vi "Copy attachment to data folder.vi"(10 "Str Refnum":refnum<vi>, 11 "Path in":refnum<vi>) -> (0 "error out":errorcluster)   [LabVIEW 2015]
uses:
  controls/Global.vi
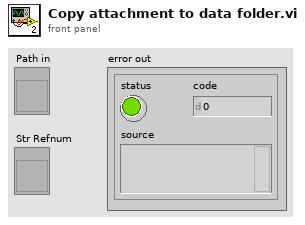
[diagram p1: front panel]
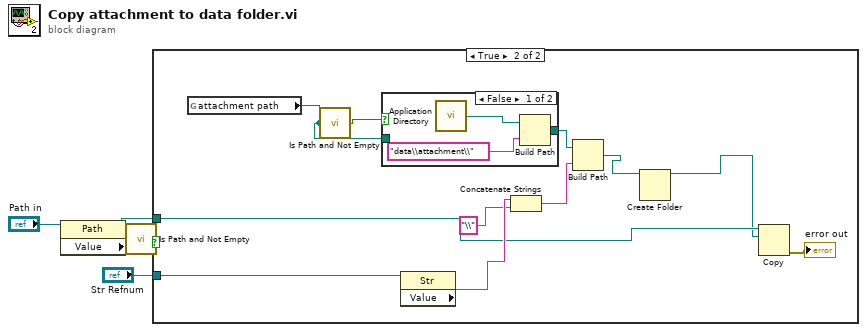
[diagram p0: block diagram]
diagram:
  n1 = property on="Property Node" class="Path"(reference="Path in") -> ("Value"=w4:path)  [unwired: 1 in, 2 out]
  n2 = call <vilib>:"Is Path and Not Empty.vi"("path"=w4) -> ("Is Path and Not Empty?"=w3:bool)  [unwired: 4 in]
  n3 = case shown="True" w3 {
    tunnel: w4 -> [_ w12]
    tunnel: "Str Refnum" -> [_ w8]
    frame False {
    }
    frame True {
      n4 = global read "Global.vi" "attachment path"() -> (w5:path)
      n5 = call <vilib>:"Is Path and Not Empty.vi"("path"=w5) -> ("Is Path and Not Empty?"=w6:bool)  [unwired: 4 in]
      n6 = case shown="False" w6 {
        tunnel: [w17 w19] -> w7
        tunnel: w5 -> [_ w19]
        frame False {
          n7 = call <vilib>:"Application Directory.vi"() -> ("Application Directory"=w18:path)
          n8 = Build Path(base path=w18, name or relative path="data\\attachment\\") -> (appended path=w17:path)
        }
        frame True {
        }
      }
      n9 = property on="Property Node" class="Str"(reference=w8) -> ("Value"=w15:string)  [unwired: 1 in, 2 out]
      n10 = Concatenate Strings(w15, "\\") -> (w13:string)
      n11 = Build Path(base path=w7, name or relative path=w13) -> (appended path=w10:path)
      n12 = Create Folder(path (use dialog)=w10) -> (created path=w9:path)  [unwired: 2 in, 2 out]
      n13 = Copy(10:w9, 11:w12) -> (0:→"error out":errorcluster)  [unwired: 3 in, 2 out]
    }
  }
